vi "Collect Case Result.vi"(10 "Test Case Result":T1, 11 "Report Generator In":refnum<class "Result Collector.lvclass">) -> (3 "Report Generator Out":refnum<class "Result Collector.lvclass">)   [LabVIEW 2020, in "Result Collector.lvclass"]
uses:
  Result Collector.lvclass
  Result Types/Case Result/Test Case Result.ctl
  Result Types/Method Result/Method Result.ctl
  Result Types/Assertion Result/Public/TypeDefs/Status.ctl
  Result Types/Assertion Result/Assertion Result.ctl
  Result Types/Assertion Result/Public/TypeDefs/Assertion Type.ctl
  Result Collector.lvclass/Result Collector.ctl
  Result Types/Assertion Result/Assertion Result.lvlib
  Result Types/Method Result/Method Result.lvlib
  Result Types/Case Result/Test Case Result.lvlib
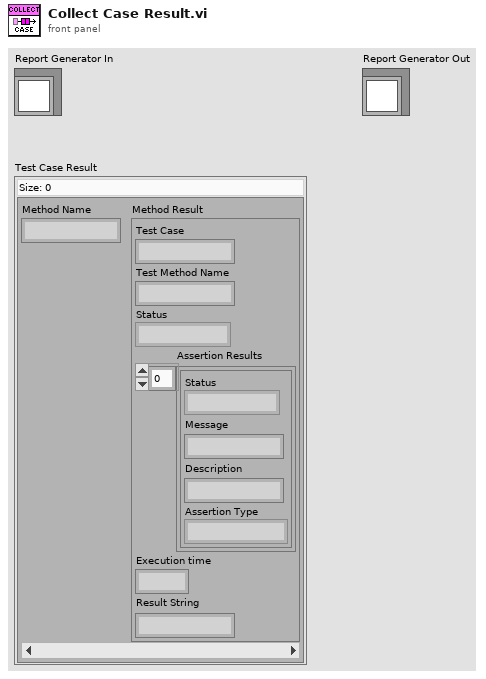
[diagram p1: front panel]
types:
  T1 = typedef "Test Case Result.lvlib/Test Case Result.ctl" = map{string, T2}
  T2 = typedef "Method Result.lvlib/Method Result.ctl" = cluster{"Test Case":string, "Test Method Name":string, "Status":T3, "Assertion Results":T4[], "Execution time":dbl, "Result String":string}
  T3 = typedef "Assertion Result.lvlib/Status.ctl" = enum16{"Pass", "Fail", "Error", "Skipped", "Setup Error", "Broken", "Teardown Error"}
  T4 = typedef "Assertion Result.lvlib/Assertion Result.ctl" = cluster{"Status":T3, "Message":string, "Description":string, "Assertion Type":T5}
  T5 = typedef "Assertion Result.lvlib/Assertion Type.ctl" = enum16{"None", "Pass", "Fail", "Skip", "Pass if Equal", "Fail if Equal", "Pass if Error", "Fail if Error", "Pass if", "Fail if"}
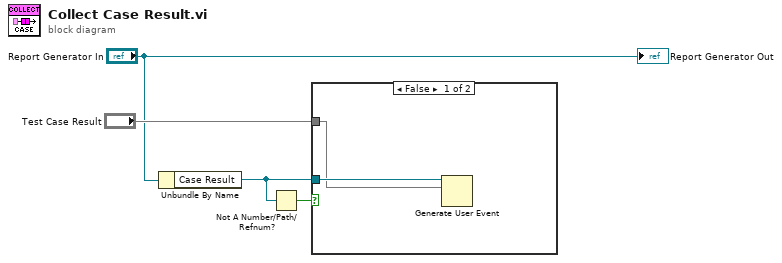
[diagram p0: block diagram]
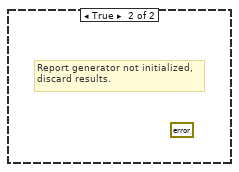
[diagram p2: hidden frame]
diagram:
  n1 = Unbundle By Name("Report Generator In") -> ("Case Result"=w3:refnum<user-event>)
  n2 = Not A Number/Path/Refnum?(number/path/refnum=w3) -> (NaN/Path/Refnum?=w4:bool)
  n3 = case shown="False" w4 {
    tunnel: "Test Case Result" -> [w5 _]
    tunnel: w3 -> [w6 _]
    frame False {
      n4 = Generate User Event(user event=w6, event data cluster=w5) -> ()  [unwired: 2 in, 2 out]
    }
    frame True {
      (unwired) errorcluster {"status"=FALSE, "code"=0, "source"=""} ("error out")
      # "Report generator not initialized,\ndiscard results."
    }
  }
  "Report Generator Out" <- "Report Generator In"
